vi "Reset Backlog Registry.vi"(8 "error in (no error)":errorcluster, 10 "TimingEngine":T1, 11 "FP Controls in":refnum<class "FP Controls.lvclass">) -> (0 "error out":errorcluster, 3 "FP Controls out":refnum<class "FP Controls.lvclass">)   [LabVIEW 2018, in "Configuration Grandmaster.lvlib" / "FP Controls.lvclass"]
uses:
  FP Controls.lvclass
  Common/Controls/TE_Designator.ctl
  FP Controls.lvclass/FP Controls.ctl
  Common/Controls/DAQ Diagnostics.ctl
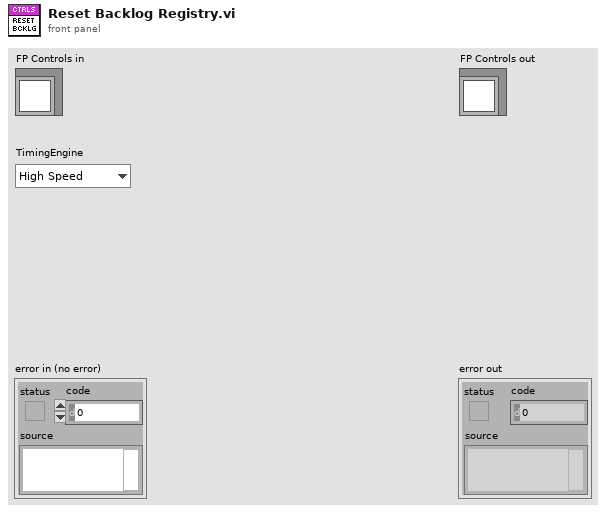
[diagram p1: front panel]
types:
  T1 = typedef "TE_Designator.ctl" = enum16{"High Speed", "Low Speed"}
  T2 = typedef "DAQ Diagnostics.ctl" = cluster{"New":bool, "LoopRate (ms)":u32, "Bff Bcklg":dbl}
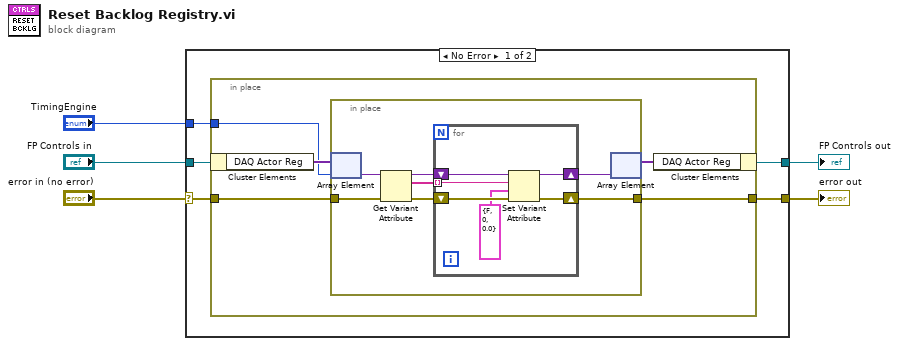
[diagram p0: block diagram]
diagram:
  n1 = case shown="No Error" "error in (no error)" {
    selector: "error in (no error)" -> [w8 w30]
    tunnel: [w6 w30] -> w4
    tunnel: [w7 w29] -> w2
    tunnel: "FP Controls in" -> [w10 w29]
    tunnel: "TimingEngine" -> [w9 _]
    frame No Error {
      n2 = in-place {
        in-place-border: w9 -> [w14]
        in-place-border: w8 -> [w13]
        in-place-border: [w11] -> w6
        n3 = in-place-cluster #1(w10) -> ("DAQ Actor Reg"=w15:variant[])
        n4 = in-place {
          in-place-border: w13 -> [w21]
          in-place-border: [w17] -> w11
          n5 = in-place-array #2(w15, w14) -> (w22:variant)
          n6 = Get Variant Attribute(Variant=w22, error in=w21) -> (duplicate Variant=w20:variant, names=w16:string[], error out=w18:errorcluster)  [unwired: 2 in, 1 out]
          n7 = for {
            shift-right: [w25] -> w19
            shift-left: w20 -> [w28]
            shift-right: [w24] -> w17
            shift-left: w18 -> [w27]
            tunnel: w16 -> [w26] mode=indexing
            n8 = Set Variant Attribute(Variant=w28, name=w26, value=T2 {"New"=FALSE, "LoopRate (ms)"=0, "Bff Bcklg"=0.0} ("DAQ Diag"), error in=w27) -> (Variant out=w25:variant, error out=w24:errorcluster)  [unwired: 1 out]
          }
          n9 = in-place-array #2(w19) -> (w12:variant[])  [unwired: 1 out]
        }
        n10 = in-place-cluster #1("DAQ Actor Reg"=w12) -> (w7:refnum<class "FP Controls.lvclass">)
      }
    }
    frame Error {
    }
  }
  "error out" <- w4
  "FP Controls out" <- w2
